vi "Test-KH_CDC_Scale_REV2.vi"(10 "Scale":dbl, 11 "r":dbl) -> (3 "2byte":dbl)   [LabVIEW 2015]
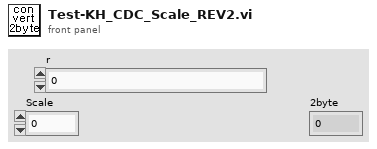
[diagram p1: front panel]
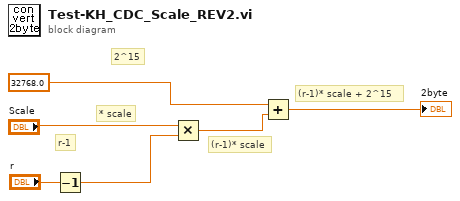
[diagram p0: block diagram]
diagram:
  # "(r-1)* scale + 2^15"
  # "(r-1)* scale"
  # "* scale"
  # "r-1"
  # "2^15"
  n1 = Decrement(x="r") -> (x-1=w6:dbl)
  n2 = Multiply(x="Scale", y=w6) -> (x*y=w5:dbl)
  n3 = Add(x=32768.0, y=w5) -> (x+y=→"2byte":dbl)
